vi "7-scan.vi"(3 "this":i32, 4 "button":i32, 5 "shift in":bool, 6 "settings in":T1={"Auto1"=TRUE, "Auto2"=TRUE, "Rel1"=TRUE, "Rel2"=TRUE, "Filt1"=TRUE, "Filt2"=TRUE, "Rate"=enum."Med", "Range1"=enum."10mV", "Range2"=enum."100mV", "Filt3"=TRUE, "Filt4"=TRUE, "Rel temp"=TRUE, "Analog1"=FALSE, "Analog2"=FALSE, "Analog temp"=FALSE, "Digital1"=TRUE, "Digital2"=TRUE, "Digital temp "=TRUE, "Window1"=enum."0,01%", "Window2"=enum."0,01%", "Window temp"=enum."0,01%", "RDGS1"="010", "RDGS2"="010", "RDGS temp"="010", "Type_type1"=TRUE, "Type_type2"=TRUE, "Type_type temp"=TRUE, "LSync"=FALSE, "Unit"=enum."C", "Sens"=TRUE, "Type tcoupl"=enum."J", "Junc"=TRUE}) -> (0 "next state":i32, 1 "shift out":bool, 2 "settings out":T1)   [LabVIEW 2017]
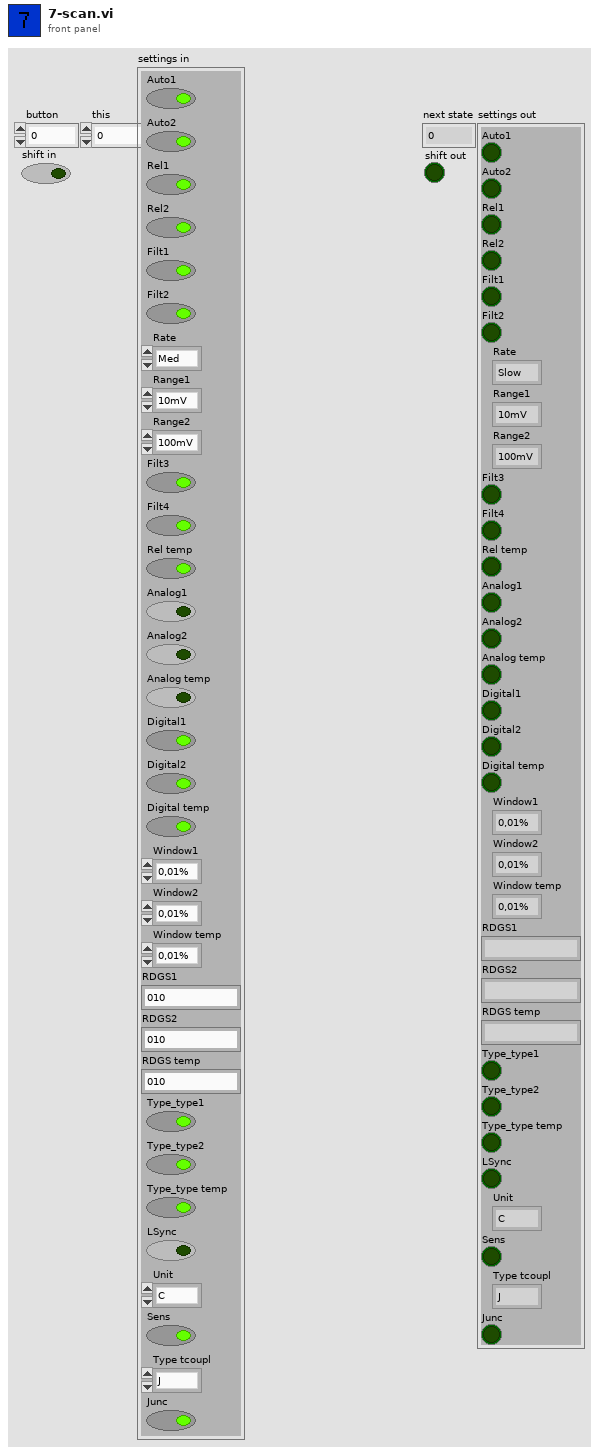
[diagram p1: front panel]
types:
  T1 = cluster{"Auto1":bool, "Auto2":bool, "Rel1":bool, "Rel2":bool, "Filt1":bool, "Filt2":bool, "Rate":enum16{"Slow", "Med", "Fast"}, "Range1":enum16{"10mV", "100mV", "1V", "10V", "100V"}, "Range2":enum16{"100mV", "1V", "10V"}, "Filt3":bool, "Filt4":bool, "Rel temp":bool, "Analog1":bool, "Analog2":bool, "Analog temp":bool, "Digital1":bool, "Digital2":bool, "Digital temp ":bool, "Window1":enum16{"0,01%", "0,1%", "1%", "10%", "None"}, "Window2":enum16{"0,01%", "0,1%", "1%", "10%", "None"}, "Window temp":enum16{"0,01%", "0,1%", "1%", "10%", "None"}, "RDGS1":string, "RDGS2":string, "RDGS temp":string, "Type_type1":bool, "Type_type2":bool, "Type_type temp":bool, "LSync":bool, "Unit":enum16{"C", "K", "F"}, "Sens":bool, "Type tcoupl":enum16{"J", "K", "T", "E", "R", "S", "B", "N"}, "Junc":bool}
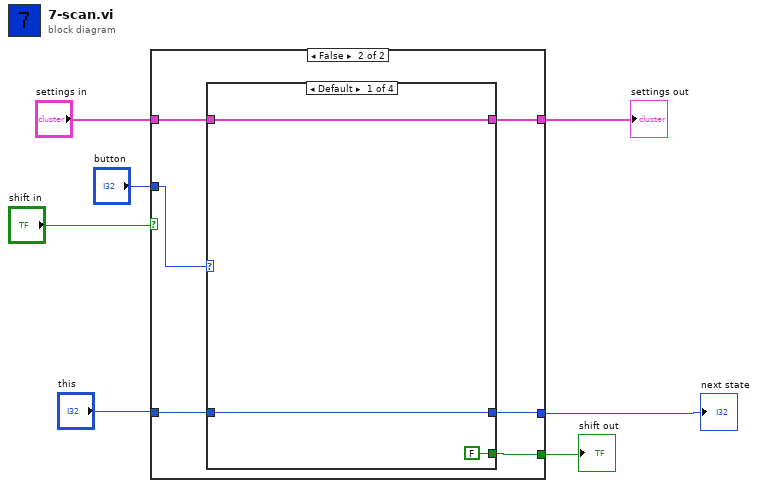
[diagram p0: block diagram]
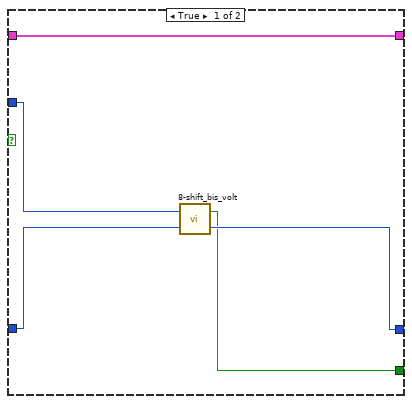
[diagram p2: hidden frame]
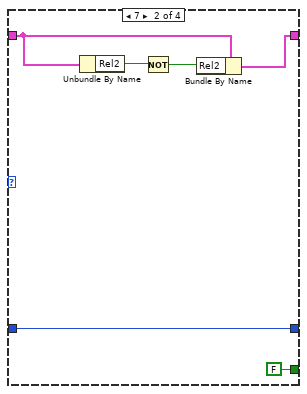
[diagram p3: hidden frame]
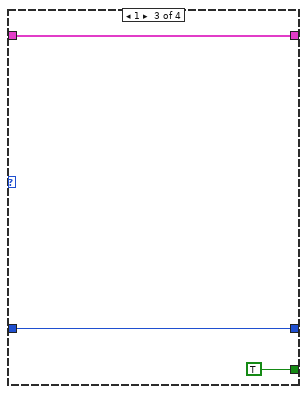
[diagram p4: hidden frame]
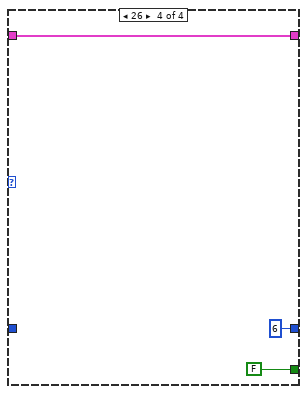
[diagram p5: hidden frame]
diagram:
  n1 = case shown="False" "shift in" {
    tunnel: "button" -> [w11 w18]
    tunnel: [w9 w15] -> w5
    tunnel: "this" -> [w10 w16]
    tunnel: [w8 w17] -> w3
    tunnel: "settings in" -> [w12 w14]
    tunnel: [w12 w13] -> w1
    frame True {
      n2 = call "8-shift_bis_volt.vi"("this"=w10, "button"=w11) -> ("next state"=w9:i32, "shift"=w8:bool)
    }
    frame False {
      n3 = case shown="Default" w18 {
        tunnel: [FALSE FALSE TRUE FALSE] -> w17
        tunnel: w16 -> [w21 w27 w29 _]
        tunnel: [w21 w27 w29 6 ("this")] -> w15
        tunnel: [w19 w23 w28 w32] -> w13
        tunnel: w14 -> [w19 w22 w28 w32]
        frame Default {
        }
        frame 7 {
          n4 = Unbundle By Name(w22) -> ("Rel2"=w25:bool)
          n5 = Not(x=w25) -> (.not. x?=w24:bool)
          n6 = Bundle By Name(cluster=w22, "Rel2"=w24) -> (w23:T1)
        }
        frame 1 {
        }
        frame 26 {
        }
      }
    }
  }
  "next state" <- w5
  "shift out" <- w3
  "settings out" <- w1
